vi "SECoP-addReadableParameter.vi"(6 "description":string, 7 "datainfo":string, 8 "error in (no error)":errorcluster, 10 "parameter name":string, 11 "DLL path (in)":T1) -> (0 "error out":errorcluster, 3 "DLL path (out)":T1)   [LabVIEW 2023, in "SECoP.lvlib"]
doc: "Call <b>\"SECoP-addReadableParameter.vi\"</b> to create a read only SECoP parameter inside the last created SECoP module.\n\n<b>DLL path</b> input and output of cluster from \"SECoP-Initialize.vi\"\n<b>parameter name</b> name of parameter\n<b>datainfo</b> data info (data type of parameter, see SECoP specification)\n<b>description</b> human readable description of this parameter"
uses:
  SECoP.lvlib
  SECoP-libraries.ctl
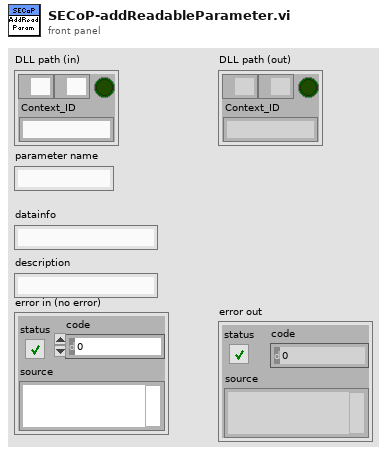
[diagram p1: front panel]
types:
  T1 = typedef "SECoP.lvlib/SECoP-libraries.ctl" = cluster{"serverDLL":path, "variantDLL":path, "cleanup_mode":bool, "Context_ID":string}
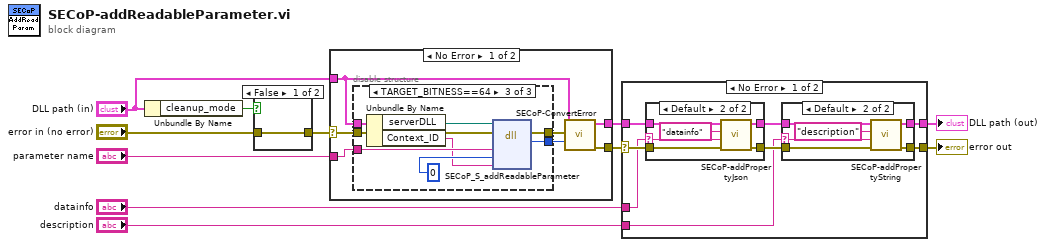
[diagram p0: block diagram]
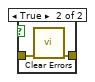
[diagram p5: hidden frame]
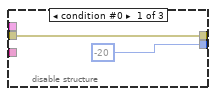
[diagram p6: hidden frame]
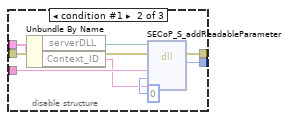
[diagram p7: hidden frame]
diagram:
  n1 = Unbundle By Name("DLL path (in)") -> ("cleanup_mode"=w10:bool)
  n2 = case shown="False" w10 {
    tunnel: "error in (no error)" -> [w12 w14]
    tunnel: [w12 w13] -> w8
    frame False {
    }
    frame True {
      n3 = call <vilib>:"Clear Errors.vi"("error in (no error)"=w14) -> ("error out"=w13:errorcluster)  [unwired: 5 in, 1 out]
    }
  }
  n4 = case shown="No Error" w8 {
    selector: w8 -> [w19 w40]
    tunnel: "DLL path (in)" -> [w15 w41]
    tunnel: [w20 w41] -> w3
    tunnel: [w21 w40] -> w4
    tunnel: "parameter name" -> [w16 _]
    frame No Error {
      n5 = disable-structure shown="TARGET_BITNESS==64" {
        disable-tunnel: w19 -> [w23 w31 w39]
        disable-tunnel: w15 -> [_ w30 w38]
        disable-tunnel: [w23 w29 w37] -> w18
        disable-tunnel: [-20 ("return type") w28 w36] -> w17
        disable-tunnel: w16 -> [_ w27 w35]
        frame condition #0 {
        }
        frame condition #1 {
          n6 = Unbundle By Name(w30) -> ("serverDLL"=w25:path, "Context_ID"=w24:string)
          n7 = dll-call lib="C:/Users/user/Desktop/x86_64/SECoP64.dll" fn="SECoP_S_addReadableParameter"(path in=w25, error in=w31, "name"=w27, "function pointer"=u32 0, "szContextID"=w24) -> (error out=w29:errorcluster, "return type"=w28:i32)  [unwired: 4 in, 1 out]
        }
        frame condition #2 (active) {
          n8 = Unbundle By Name(w38) -> ("serverDLL"=w33:path, "Context_ID"=w32:string)
          n9 = dll-call lib="C:/Users/user/Desktop/x86_64/SECoP64.dll" fn="SECoP_S_addReadableParameter"(path in=w33, error in=w39, "name"=w35, "function pointer"=u64 0, "szContextID"=w32) -> (error out=w37:errorcluster, "return type"=w36:i32)  [unwired: 4 in, 1 out]
        }
      }
      n10 = call "SECoP-ConvertError.vi"("return code"=w17, "error in (no error)"=w18, "DLL path (in)"=w15) -> ("error out"=w21:errorcluster, "DLL path (out)"=w20:T1)  [unwired: 7 in]
    }
    frame Error {
    }
  }
  n11 = case shown="No Error" w4 {
    selector: w4 -> [w47 w67]
    tunnel: w3 -> [w48 w66]
    tunnel: [w42 w67] -> w1
    tunnel: [w43 w66] -> w2
    tunnel: "datainfo" -> [w46 _]
    tunnel: "description" -> [w45 _]
    frame No Error {
      n12 = case shown="Default" w46 {
        selector: w46 -> [_ w61]
        tunnel: w48 -> [w59 w65]
        tunnel: w47 -> [w58 w64]
        tunnel: [w58 w63] -> w49
        tunnel: [w59 w62] -> w44
        frame "" {
        }
        frame Default {
          n13 = call "SECoP-addPropertyJson.vi"("error in (no error)"=w64, "property value"=w61, "property name"="datainfo", "DLL path (in)"=w65) -> ("error out"=w63:errorcluster, "DLL path (out)"=w62:T1)  [unwired: 6 in]
        }
      }
      n14 = case shown="Default" w45 {
        selector: w45 -> [_ w53]
        tunnel: w44 -> [w51 w57]
        tunnel: w49 -> [w50 w56]
        tunnel: [w50 w55] -> w42
        tunnel: [w51 w54] -> w43
        frame "" {
        }
        frame Default {
          n15 = call "SECoP-addPropertyString.vi"("error in (no error)"=w56, "property value"=w53, "property name"="description", "DLL path (in)"=w57) -> ("error out"=w55:errorcluster, "DLL path (out)"=w54:T1)  [unwired: 6 in]
        }
      }
    }
    frame Error {
    }
  }
  "DLL path (out)" <- w2
  "error out" <- w1
